vi "FABR-Synthesize Waveforms.vi"(0 "SC":T2, 5 "Runtime in":T1) -> (4 "Stim":dbl[](array[numeric]))   [LabVIEW 2020]
uses:
  Typedefs/FABR-Stimulus Condition.ctl
  Typedefs/FABR-Runtime Data.ctl
  <vilib>/Analysis/NI_AALBase.lvlib
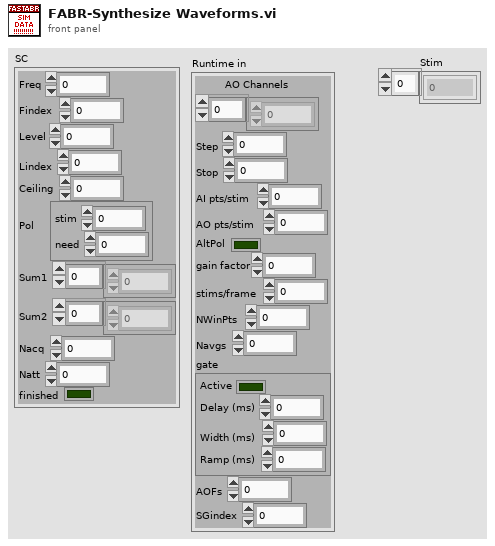
[diagram p1: front panel]
types:
  T1 = typedef "FABR-Runtime Data.ctl" = cluster{"AO Channels":i32[], "Step":dbl, "Stop":i32, "AI pts/stim":i32, "AO pts/stim":i32, "AltPol":bool, "gain factor":dbl, "stims/frame":i32, "NWinPts":i32, "Navgs":i32, "gate":cluster{"Active":bool, "Delay (ms)":dbl, "Width (ms)":dbl, "Ramp (ms)":dbl}, "AOFs":dbl, "SGindex":i32}
  T2 = typedef "FABR-Stimulus Condition.ctl" = cluster{"Freq":dbl, "Findex":i32, "Level":dbl, "Lindex":i32, "Ceiling":dbl, "Pol":cluster{"stim":i32, "need":i32}, "Sum1":dbl[], "Sum2":dbl[], "Nacq":i32, "Natt":i32, "finished":bool}
  T3 = cluster{"Active":bool, "Delay (ms)":dbl, "Width (ms)":dbl, "Ramp (ms)":dbl}
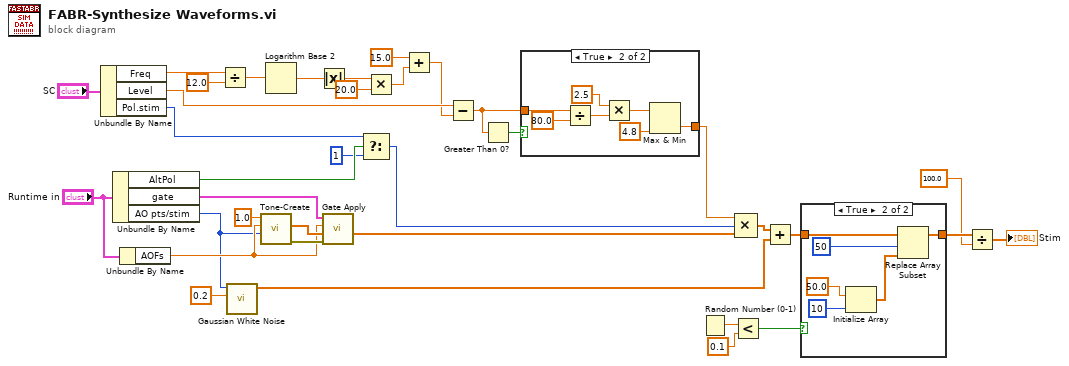
[diagram p0: block diagram]
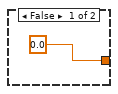
[diagram p3: hidden frame]
diagram:
  n1 = Unbundle By Name("SC") -> ("Freq"=w30:dbl, "Level"=w19:dbl, "Pol.stim"=w2:i32)
  n2 = Unbundle By Name("Runtime in") -> ("AltPol"=w4:bool, "gate"=w33:T3, "AO pts/stim"=w20:i32)
  n3 = Unbundle By Name("Runtime in") -> ("AOFs"=w32:dbl)
  n4 = Divide(x=w30, y=12.0) -> (x/y=w28:dbl)
  n5 = call <vilib>:"Gaussian White Noise.vi"("standard deviation"=0.2, "samples"=w20) -> ("Gaussian noise pattern"=w13:dbl[])  [unwired: 8 in, 1 out]
  n6 = call "Tone-Create.vi"("Npts"=w20, "Sampling Rate (Hz)"=w32, "Frequency (kHz)"=1.0) -> ("error out"=w36:errorcluster, "Waveform"=w35:dbl[])  [unwired: 7 in]
  n7 = Logarithm Base 2(1:w28) -> (0:w26:dbl)
  n8 = Absolute Value(x=w26) -> (abs(x)=w25:dbl)
  n9 = call "Gate Apply.vi"("error in (no error)"=w36, "Waveform in"=w35, "Sampling Rate (Hz)"=w32, "Gate Control"=w33) -> ("Gated waveform"=w15:dbl[])  [unwired: 6 in, 1 out]
  n10 = Select(t=w2, s=w4, f=1 ("t")) -> (s? t:f=w3:i32)
  n11 = Multiply(x=w25, y=20.0) -> (x*y=w22:dbl)
  n12 = Add(x=15.0, y=w22) -> (x+y=w18:dbl)
  n13 = Subtract(x=w19, y=w18) -> (x-y=w16:dbl)
  n14 = Greater Than 0?(x=w16) -> (x > 0?=w17:bool)
  n15 = case shown="True" w17 {
    tunnel: w16 -> [_ w44]
    tunnel: [0.0 w38] -> w5
    frame False {
    }
    frame True {
      n16 = Divide(x=w44, y=80.0) -> (x/y=w42:dbl)
      n17 = Multiply(x=2.5, y=w42) -> (x*y=w40:dbl)
      n18 = Max & Min(x=w40, y=4.8) -> (min(x,y)=w38:dbl)  [unwired: 1 out]
    }
  }
  n19 = Random Number (0-1)() -> (number: 0 to 1=w11:dbl)
  n20 = Less?(x=w11, y=0.1) -> (x < y?=w8:bool)
  n21 = Compound Arithmetic op=MULTIPLY(w5, w3, w15) -> (w14:dbl[])
  n22 = Add(x=w14, y=w13) -> (x+y=w9:dbl[])
  n23 = case shown="True" w8 {
    tunnel: w9 -> [w45 w51]
    tunnel: [w45 w50] -> w7
    frame False {
    }
    frame True {
      n24 = Initialize Array(50.0 ("new element/subarray"), 10 ("dimension size")) -> (w46:dbl[])
      n25 = Replace Array Subset(array=w51, new element=w46, index=50) -> (w50:dbl[])
    }
  }
  n26 = Divide(x=w7, y=100.0) -> (x/y=→"Stim":dbl[])
